vi "GUI_001.vi"(2 "Numeric":dbl) -> (0 "Slide":dbl(slide) scale=0.0..100.0)   [LabVIEW 2019]
panel:
  out "Waveform Chart":dbl(graph)
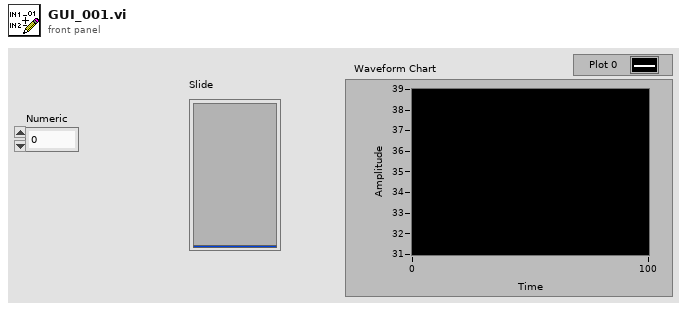
[diagram p1: front panel]
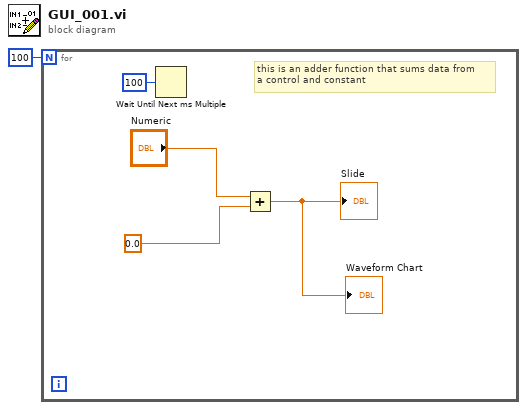
[diagram p0: block diagram]
diagram:
  n1 = for {
    N: 100 -> [_]
    # "this is an adder function that sums data from\na control and constant"
    n2 = Wait Until Next ms Multiple(millisecond multiple=u32 100) -> ()  [unwired: 1 out]
    n3 = Add(x="Numeric", y=0.0) -> (x+y=→"Slide" →"Waveform Chart":dbl)
  }
